vi "test_Teardown_Testenvironment.vi"(8 "error in":errorcluster, 11 "GenericDevice.lvclass":refnum<class "GenericDevice.lvclass">) -> (0 "error out":errorcluster, 2 "device is open?":bool)   [LabVIEW 2023]
uses:
  Source/Classes/GenericDevice/GenericDevice.lvclass
  Source/Libraries/DeviceManager/DeviceManager.lvlib
panel:
  # "Connector Pane"
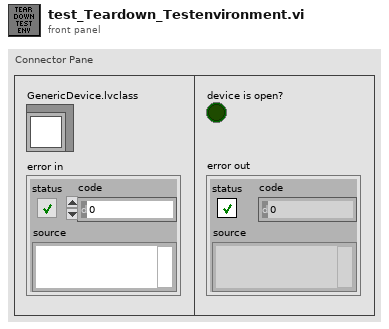
[diagram p1: front panel]
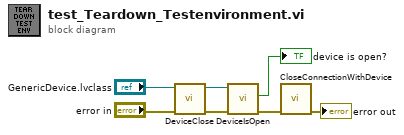
[diagram p0: block diagram]
diagram:
  n1 = call-dynamic "DeviceClose.vi"("error in (no error)"="error in", "GenericDevice in"="GenericDevice.lvclass") -> ("error out"=w5:errorcluster, "GenericDevice out"=w6:refnum<class "GenericDevice.lvclass">)  [unwired: 5 in, 3 out]
  n2 = call-dynamic "DeviceIsOpen.vi"("error in (no error)"=w5, "GenericDevice in"=w6) -> ("error out"=w4:errorcluster, "device is open?"=→"device is open?":bool)  [unwired: 6 in, 2 out]
  n3 = call "CloseConnectionWithDevice.vi"("error in (no error)"=w4) -> ("error out"=→"error out":errorcluster)  [unwired: 10 in]
